vi "measurementInputPanel.vi"() -> ()   [LabVIEW 2013]
uses:
  Controls/instruType.ctl
  Controls/sigProcessType.ctl
panel:
  out "?":T3(array[cluster]) {"Instru Type" items=["Raw voltage", "Pressure Scanner", "Pressure Transducer", "Pitot-static Tube", "13-Hole Probe"]}
  in  "Acquisition Cards":u16(ring) items=["NI-USB-6210_Kernel.vi"]
  in  "Setup":enum16{"Run Programme", "Show Setup"}(ring)
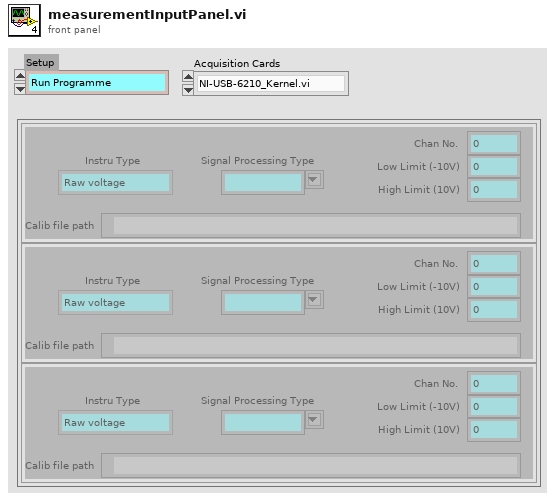
[diagram p1: front panel]
types:
  T1 = typedef "instruType.ctl" = u16
  T2 = typedef "sigProcessType.ctl" = string
  T3 = cluster{"Low Limit (-10V)":dbl, "High Limit (10V)":dbl, "Chan No.":i32, "Calib file path":path, "Instru Type":T1, "Signal Processing Type":T2}[]
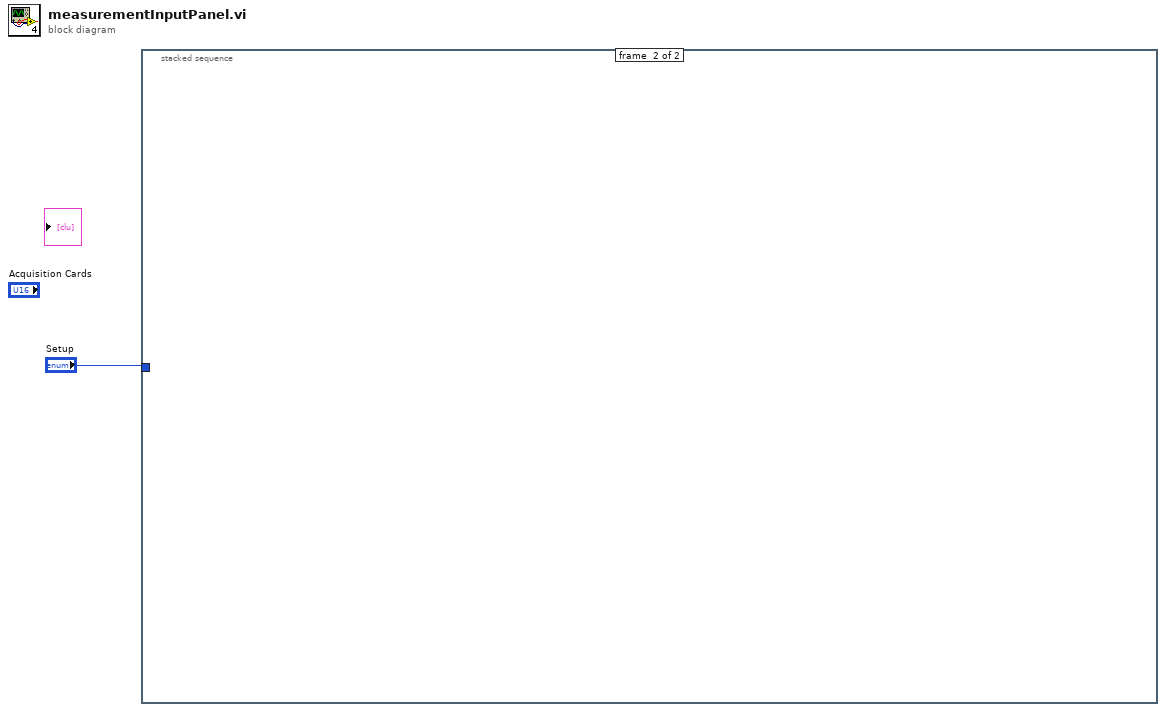
[diagram p0: block diagram]
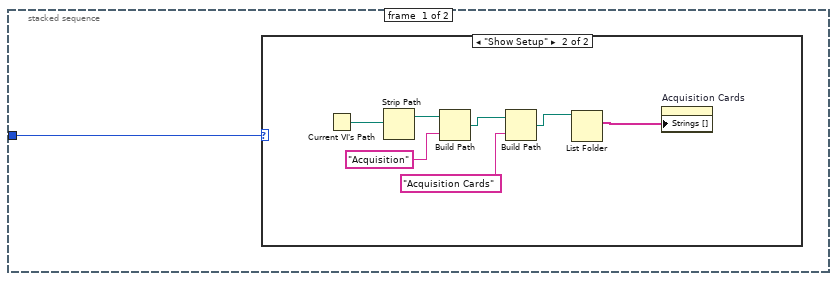
[diagram p2: hidden frame]
diagram:
  n1 = stacked-sequence {
    tunnel: "Setup" -> [w2 _]
    frame #0 {
      n2 = case shown="\"Show Setup\"" w2 {
        frame "Run Programme", Default {
        }
        frame "Show Setup" {
          n3 = Current VI's Path() -> (path=w9:path)
          n4 = Strip Path(path=w9) -> (stripped path=w8:path)  [unwired: 1 out]
          n5 = Build Path(base path=w8, name or relative path="Acquisition") -> (appended path=w6:path)
          n6 = Build Path(base path=w6, name or relative path="Acquisition Cards") -> (appended path=w4:path)
          n7 = List Folder(path=w4) -> (filenames=w3:string[])  [unwired: 3 in, 3 out]
          n8 = property on="Acquisition Cards" class="Ring (strict)"("Strings []"=w3) -> ()  [unwired: 2 in, 2 out]
        }
      }
    }
    frame #1 {
    }
  }
